vi "Parse Table Names.vi"(8 "error in (no error)":errorcluster, 10 "start at":i32, 11 "TOML String":string) -> (0 "error out":errorcluster, 2 "offset past match":i32, 3 "Table Stack":string[](array[string]))   [LabVIEW 2019, in "BlueTOMLSerializer.lvlib"]
uses:
  BlueTOMLSerializer.lvlib
  <vilib>/regexp/Match Regular Expression.xnode
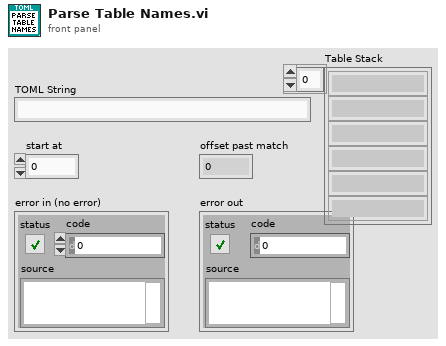
[diagram p1: front panel]
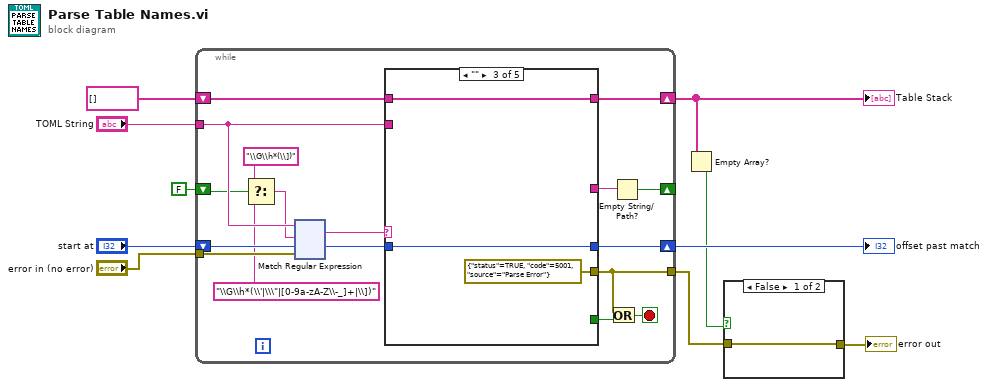
[diagram p0: block diagram]
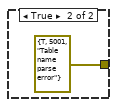
[diagram p2: hidden frame]
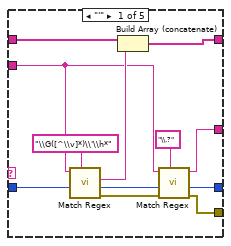
[diagram p3: hidden frame]
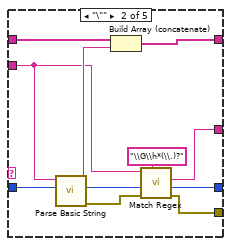
[diagram p4: hidden frame]
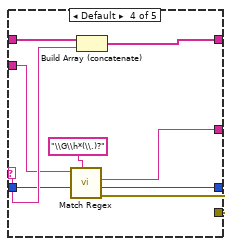
[diagram p5: hidden frame]
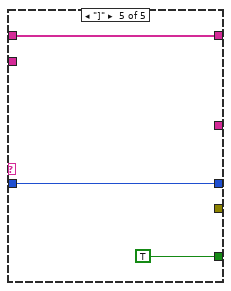
[diagram p6: hidden frame]
diagram:
  n1 = while {
    tunnel: "error in (no error)" -> [w27]
    tunnel: "TOML String" -> [w23]
    shift-right: [w21] -> w6
    shift-left: "start at" -> [w26]
    tunnel: [w17] -> w3
    shift-right: [w19] -> w5
    shift-left: string[] [] -> [w20]
    shift-right: [w15] -> _
    shift-left: FALSE -> [w14]
    stop <- w25 stop-if-true
    n2 = Select(t="\\G\\h*(\\])" ("regular expression"), s=w14, f="\\G\\h*(\\'|\\\"|[0-9a-zA-Z\\-_]+|\\])" ("regular expression")) -> (s? t:f=w13:string)
    n3 = xnode "Match Regular Expression"("input string"=w23, "regular expression"=w13, "offset (0)"=w26, "error in"=w27) -> ("whole match"=w24:string, "offset past match"=w22:i32)  [unwired: 2 in, 3 out]
    n4 = case shown="\"\"" w24 {
      selector: w24 -> [_ _ _ w62 _]
      tunnel: [w31 w42 w52 w57 w65] -> w21
      tunnel: w22 -> [w36 w50 w52 w58 w65]
      tunnel: [w28 w43 errorcluster {"status"=TRUE, "code"=5001, "source"="Parse Error"} ("error constant") w56 _] -> w17
      tunnel: w23 -> [w33 w44 _ w59 _]
      tunnel: w20 -> [w39 w49 w51 w61 w64]
      tunnel: [w38 w41 w51 w55 w64] -> w19
      tunnel: [_ _ _ _ TRUE] -> w18
      tunnel: [w30 w40 _ w54 _] -> w16
      frame "'" {
        n5 = call "Match Regex.vi"("regular expression"="\\G([^\\v]*)\\'\\h*", "offset"=w36, "String"=w33) -> ("error out"=w29:errorcluster, "offset past match"=w34:i32, "submatch 1"=w35:string)  [unwired: 5 in, 1 out]
        n6 = Build Array (concatenate)(w39, w35) -> (w38:string[])
        n7 = call "Match Regex.vi"("regular expression"="\\.?", "error in (no error)"=w29, "offset"=w34, "String"=w33) -> ("error out"=w28:errorcluster, "offset past match"=w31:i32, "whole match"=w30:string)  [unwired: 4 in, 1 out]
      }
      frame "\"" {
        n8 = call "Parse Basic String.vi"("start at"=w50, "TOML String"=w44) -> ("error out"=w45:errorcluster, "offset past match"=w46:i32, "String"=w48:string)  [unwired: 7 in]
        n9 = Build Array (concatenate)(w49, w48) -> (w41:string[])
        n10 = call "Match Regex.vi"("regular expression"="\\G\\h*(\\.)?", "error in (no error)"=w45, "offset"=w46, "String"=w44) -> ("error out"=w43:errorcluster, "offset past match"=w42:i32, "submatch 1"=w40:string)  [unwired: 4 in, 1 out]
      }
      frame "" {
      }
      frame Default {
        n11 = call "Match Regex.vi"("regular expression"="\\G\\h*(\\.)?", "offset"=w58, "String"=w59) -> ("error out"=w56:errorcluster, "offset past match"=w57:i32, "submatch 1"=w54:string)  [unwired: 5 in, 1 out]
        n12 = Build Array (concatenate)(w61, w62) -> (w55:string[])
      }
      frame "]" {
      }
    }
    n13 = Or(x=w17, y=w18) -> (x .or. y?=w25:bool)
    n14 = Empty String/Path?(string/path=w16) -> (empty?=w15:bool)
  }
  "offset past match" <- w6
  "Table Stack" <- w5
  n15 = Empty Array?(array=w5) -> (empty?=w4:bool)
  n16 = case shown="False" w4 {
    tunnel: [w180 errorcluster {"status"=TRUE, "code"=5001, "source"="Table name parse error"} ("error constant")] -> w2
    tunnel: w3 -> [w180 _]
    frame False {
    }
    frame True {
    }
  }
  "error out" <- w2
